vi "MongoDB.Parse.CommandResult.vi"(8 "error in (no error)":errorcluster, 11 "MongoDB.Command.Result":refnum<k24>) -> (0 "error out":errorcluster)   [LabVIEW 2014]
uses:
  C:/Users/Richard/Documents/GitHub/mongo-labview-driver/CSharp/bin/MongoDB.Driver.Legacy.dll
  CSharp/bin/MongoDB.Driver.Legacy.dll
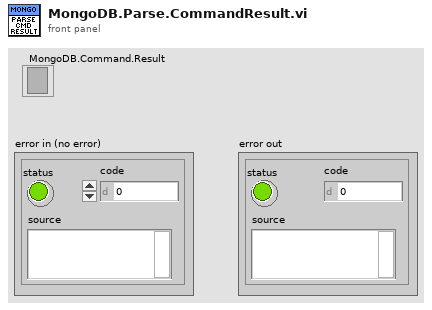
[diagram p1: front panel]
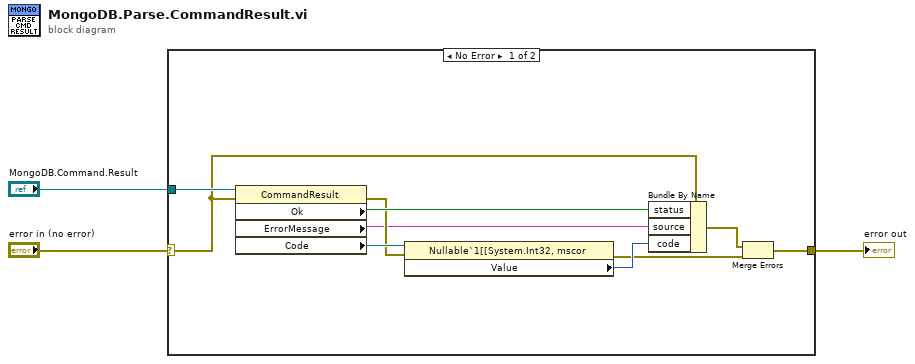
[diagram p0: block diagram]
diagram:
  n1 = case shown="No Error" "error in (no error)" {
    selector: "error in (no error)" -> [w4 w14]
    tunnel: "MongoDB.Command.Result" -> [w13 _]
    tunnel: [w5 w14] -> w2
    frame No Error {
      n2 = property class="CommandResult"(reference=w13, error in=w4) -> (error out=w10:errorcluster, "Ok"=w12:bool, "ErrorMessage"=w8:string, "Code"=w11:refnum<k24>)  [unwired: 1 out]
      n3 = property class="Nullable`1[[System.Int32, mscor"(reference=w11, error in=w10) -> (error out=w6:errorcluster, "Value"=w9:i32)  [unwired: 1 out]
      n4 = Bundle By Name(cluster=w4, "status"=w12, "source"=w8, "code"=w9) -> (w7:errorcluster)
      n5 = Merge Errors(w7, w6) -> (w5:errorcluster)
    }
    frame Error {
    }
  }
  "error out" <- w2
